vi "H036 Harsh Pandit SCADA Lab 7a Sem 6.vi"() -> ()   [LabVIEW 2018]
panel:
  out "LED Output":T1
  in  "Cluster 2":T2
  in  "Cluster 1":T3
  # "Experiment 7a: Create a VI to compare cluster 1 with numeric integer element with cluster 2 \n10 numeric integer element. Output cluster consist of 10 LEDs. Switch on the led if nth element\nof cluster 1 is more than nth element of cluster 2."
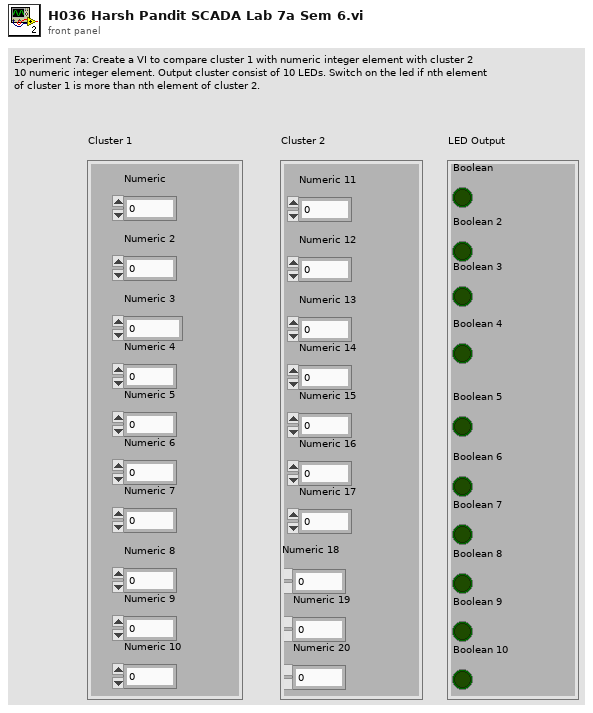
[diagram p1: front panel]
types:
  T1 = cluster{"Boolean":bool, "Boolean 2":bool, "Boolean 3":bool, "Boolean 4":bool, "Boolean 5":bool, "Boolean 6":bool, "Boolean 7":bool, "Boolean 8":bool, "Boolean 9":bool, "Boolean 10":bool}
  T2 = cluster{"Numeric 11":dbl, "Numeric 12":dbl, "Numeric 13":dbl, "Numeric 14":dbl, "Numeric 15":dbl, "Numeric 16":dbl, "Numeric 17":dbl, "Numeric 18":dbl, "Numeric 19":dbl, "Numeric 20":dbl}
  T3 = cluster{"Numeric":dbl, "Numeric 2":dbl, "Numeric 3":dbl, "Numeric 4":dbl, "Numeric 5":dbl, "Numeric 6":dbl, "Numeric 7":dbl, "Numeric 8":dbl, "Numeric 9":dbl, "Numeric 10":dbl}
  T4 = cluster{bool, bool, bool, bool, bool, bool, bool, bool, bool, bool}
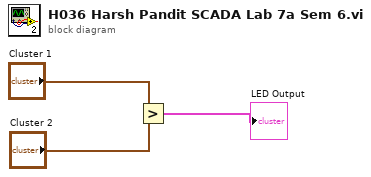
[diagram p0: block diagram]
diagram:
  n1 = Greater?(x="Cluster 1", y="Cluster 2") -> (0:→"LED Output":T4)
